vi "Untitled 1.vi"() -> ()   [LabVIEW 2016]
panel:
  out "error out":errorcluster
  out "Ingessi 2":variant
  out "Numeric":i32
  in  "milliseconds to wait":u32
  in  "stop":bool
  out "Ingessi":variant
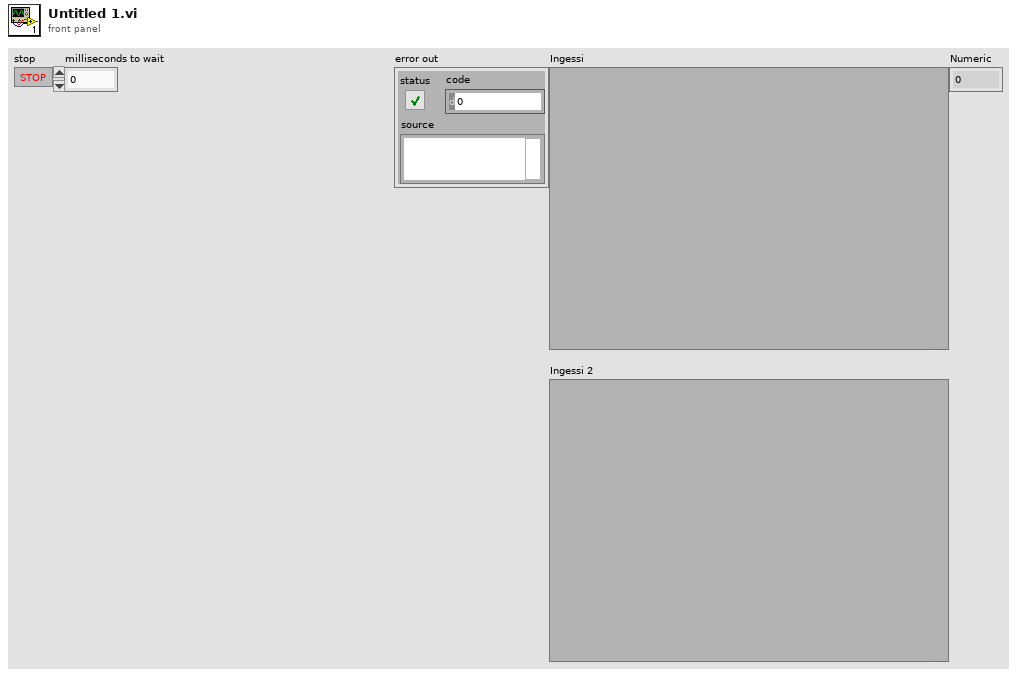
[diagram p1: front panel]
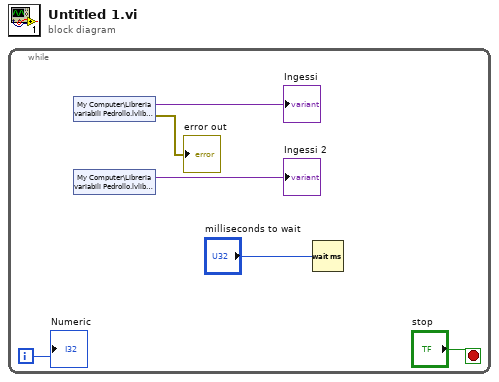
[diagram p0: block diagram]
diagram:
  n1 = while {
    i -> [w3]
    stop <- "stop" stop-if-true
    n2 = shared-variable "My Computer\\Libreria variabili Pedrollo.lvlib\\Letture"() -> (→"Ingessi":variant, error out=→"error out":errorcluster)  [unwired: 1 in]
    n3 = shared-variable "My Computer\\Libreria variabili Pedrollo.lvlib\\Letture"() -> (→"Ingessi 2":variant)  [unwired: 1 in, 1 out]
    n4 = Wait (ms)(milliseconds to wait="milliseconds to wait") -> ()  [unwired: 1 out]
    "Numeric" <- w3
  }
